vi "StartServerVi.vi"(0 "ROS in":T1={"topic port"=0, "Node"="", "topic"="", "type"="", "node port"=0, "error "={"status"=FALSE, "code"=0, "source"=""}, "Direction"=enum."Node", "APIs"=[], "Update (ms)"=1, "write queue"=1}) -> (1 "ROS out":T1={"topic port"=0, "Node"="", "topic"="", "type"="", "node port"=0, "error "={"status"=FALSE, "code"=0, "source"=""}, "Direction"=enum."Node", "APIs"=[], "Update (ms)"=1, "write queue"=1}, 2 "Reply":string, 3 "Running?":bool, 4 "error out":errorcluster)   [LabVIEW 2012]
doc: "Start a server VI for the topic. If the exists, open it. If it's running, do nothing. If it doesn't exist, create it by copying the blank server and renaming the VI."
uses:
  <userlib>/ROSforLV/ROS/Code/SubVIs/_ROSControl.ctl
  <userlib>/ROSforLV/ROS/Code/SubVIs/_ROSDirection.ctl
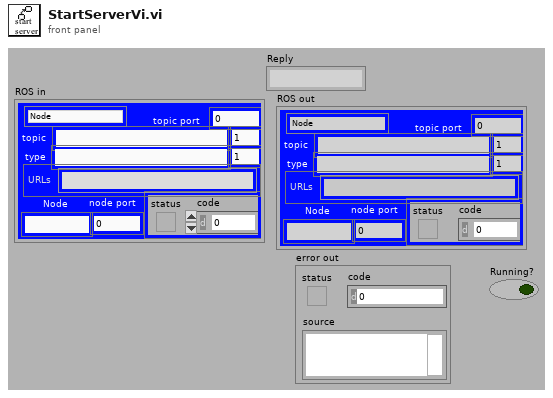
[diagram p1: front panel]
types:
  T1 = typedef "_ROSControl.ctl" = cluster{"topic port":u16, "Node":string, "topic":string, "type":string, "node port":u16, "error ":errorcluster, "Direction":T2, "APIs":string[], "Update (ms)":u16, "write queue":u16}
  T2 = typedef "_ROSDirection.ctl" = enum16{"Node", "Publisher", "Subscriber", "Service Client"}
  T3 = typedef "ServoInfo.ctl" = cluster{"vi name":string, "VI Refnum":refnum<vi>, "queue":refnum<queue>, "ROS":T1, "notifier":refnum<notifier>}
  T4 = enum32{"Bad", "Idle", "Run top level", "Running"}
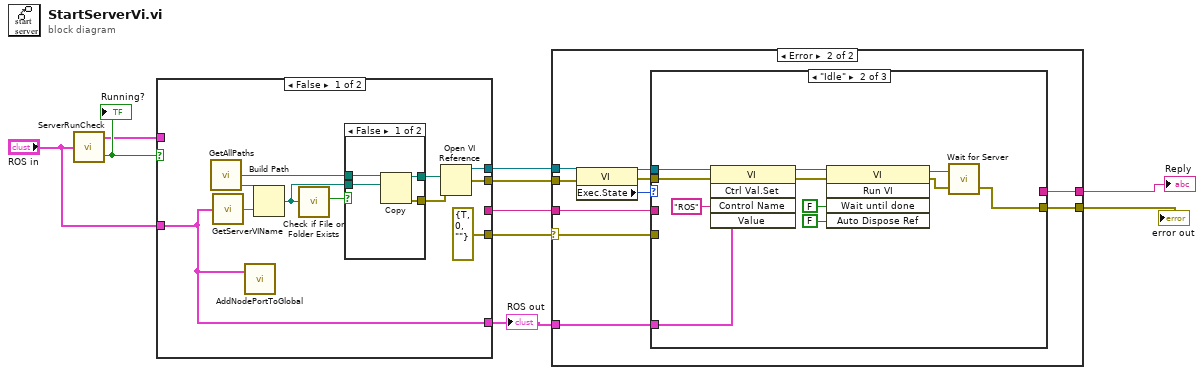
[diagram p0: block diagram]
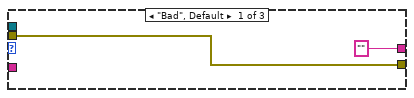
[diagram p3: hidden frame]
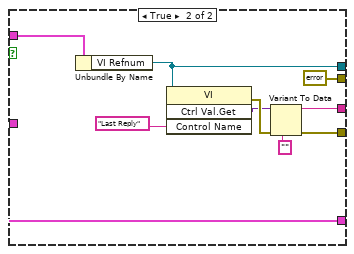
[diagram p6: hidden frame]
diagram:
  n1 = call <userlib>:"ServerRunCheck.vi"("ROS in"="ROS in") -> ("Running?"=w6:bool, "ServerFound"=w5:T3)
  "Running?" <- w6
  n2 = case shown="False" w6 {
    tunnel: [w21 w31] -> w9
    tunnel: [w20 errorcluster {"status"=FALSE, "code"=0, "source"=""} ("error out")] -> w8
    tunnel: w5 -> [_ w35]
    tunnel: "ROS in" -> [w11 w27]
    tunnel: [_ w29] -> w4
    tunnel: [errorcluster {"status"=TRUE, "code"=0, "source"=""} ("error out") w28] -> w3
    tunnel: [w11 w27] -> w1
    frame False {
      n3 = call <userlib>:"GetAllPaths.vi"() -> ("Server Folder"=w15:path, "BlankServer"=w16:path)  [unwired: 1 in, 1 out]
      n4 = call <userlib>:"GetServerVIName.vi"("ROS"=w11) -> ("vi name"=w14:string)
      n5 = call <userlib>:"AddNodePortToGlobal.vi"("ROS in"=w11) -> ()  [unwired: 3 in]
      n6 = Build Path(base path=w15, name or relative path=w14) -> (appended path=w18:path)
      n7 = call <vilib>:"Check if File or Folder Exists.vi"("path"=w18) -> ("file or folder exists?"=w17:bool)  [unwired: 8 in, 2 out]
      n8 = case shown="False" w17 {
        tunnel: w16 -> [w25 _]
        tunnel: w18 -> [w24 w26]
        tunnel: [w23 w26] -> w19
        tunnel: [w22 _] -> w12
        frame False {
          n9 = Copy(10:w24, 11:w25) -> (0:w22:errorcluster, 3:w23:path)  [unwired: 3 in, 1 out]
        }
        frame True {
        }
      }
      n10 = Open VI Reference(vi path=w19, error in (no error)=w12) -> (vi reference=w21:refnum<vi>, error out=w20:errorcluster)  [unwired: 4 in]
    }
    frame True {
      n11 = Unbundle By Name(w35) -> ("VI Refnum"=w31:refnum<vi>)
      n12 = invoke class="VI" method="Ctrl Val.Get"(reference=w31, "Control Name"="Last Reply") -> (error out=w34:errorcluster, "Get Control Value Variant"=w32:variant)  [unwired: 2 in, 2 out]
      n13 = Variant To Data(error in=w34, type="" ("Control Name"), Variant=w32) -> (data=w29:string, error out=w28:errorcluster)
    }
  }
  "ROS out" <- w1
  n14 = case shown="Error" w3 {
    selector: w3 -> [w37 w39]
    tunnel: [w38 w48] -> w10
    tunnel: w9 -> [_ w47]
    tunnel: w8 -> [_ w46]
    tunnel: [w37 w42] -> w7
    tunnel: w1 -> [_ w40]
    tunnel: w4 -> [w38 w41]
    frame No Error {
    }
    frame Error {
      n15 = property class="VI"(reference=w47, error in=w46) -> (reference out=w44:refnum<vi>, error out=w43:errorcluster, "Exec.State"=w45:T4)
      n16 = case shown="\"Idle\"" w45 {
        tunnel: w44 -> [_ w59 _]
        tunnel: [w50 w51 w62] -> w42
        tunnel: w43 -> [w50 w56 _]
        tunnel: w40 -> [_ w52 _]
        tunnel: ["" ("Control Name") _ w63] -> w48
        tunnel: w41 -> [_ _ w63]
        tunnel: w39 -> [_ _ w62]
        frame "Bad", Default {
        }
        frame "Idle" {
          n17 = invoke class="VI" method="Ctrl Val.Set"(reference=w59, error in=w56, "Control Name"="ROS", "Value"=w52) -> (reference out=w58:refnum<vi>, error out=w53:errorcluster)  [unwired: 1 in, 3 out]
          n18 = invoke class="VI" method="Run VI"(reference=w58, error in=w53, "Wait until done"=FALSE ("Wait Until Done"), "Auto Dispose Ref"=FALSE ("Wait Until Done")) -> (reference out=w54:refnum<vi>, error out=w55:errorcluster)  [unwired: 1 in, 3 out]
          n19 = call <userlib>:"Wait for Server.vi"("error in"=w55, "vi reference in"=w54) -> ("error out"=w51:errorcluster)  [unwired: 1 out]
        }
        frame "Run top level", "Running" {
        }
      }
    }
  }
  "Reply" <- w10
  "error out" <- w7
